vi "wavefront correction DMD control.vi"() -> ()   [LabVIEW 2016]
uses:
  <vilib>/DAQmx/write.llb/DAQmx Write (Analog DBL 1Chan 1Samp).vi
  <vilib>/DAQmx/read.llb/DAQmx Read (Analog 1D DBL 1Chan NSamp).vi
  <vilib>/Analysis/baseanly.llb/Mean (DBL).vi
  <vilib>/DAQmx/miscellaneous.llb/DAQmx Fill In Error Info.vi
  <vilib>/Analysis/NI_AALBase.lvlib
panel:
  out "Array":dbl[](array[numeric])
  out "1":dbl
  out "2":dbl
  out "3":dbl
  out "diff sq 3":dbl
  out "sum sq 3":dbl
  out "diff sq 2":dbl
  out "sq sum 2":dbl
  out "sum sq 1":dbl
  out "diff sq 1":dbl
  in  "t":dbl format="%#_13g"
  in  "Ignore \nthis mode":bool
  in  "Image Processing Methods":u16(ring) items=["mean", "Max Value", "sum of square", "diff square unit", "diff square"]
  out "WC finished":bool
  out "Project twice":bool
  out "Raw Data":dbl[](graph)
  out "evaluation value":dbl[](array[numeric])
  out "max index":i32
  in  "Y-Z Plane":bool
  out "Zernike index":i32
  in  "Num of Zernike Modes":dbl=3.0
  out "Real time Centre A":dbl=1.0
  out "Real time search gap":dbl
  out "unsigned 8bit integer":u8[][](array[numeric])
  out "Total Pack":dbl=6.0
  out "Hill-climbing \n   finished":bool
  in  "Ending search gap":dbl=0.05
  out "Zernike Coefficient":dbl[](array[numeric])=[0.0, 0.0, 1.0, 0.0, 0.0, 0.0, 0.0, 0.0, 0.0, 0.0, 0.0]
  in  "Start Centre A":dbl
  in  "Start search gap":dbl=0.4
  out "mean 2":dbl format="%0.2f"
  out "After oversampling-average 2":dbl[](graph)
  out "min value 2":dbl
  out "max value 2":dbl
  out "mean 1":dbl=-0.00018088652505750976 format="%0.2f"
  out "After oversampling-average 1":dbl[](graph)=[-0.0001987272925039077, -0.00015036376606842504, -0.00015036376637934116, -0.00017454552963234145, -0.0002551514075879374, -0.0001302122972688334, -0.00021887876244739687, -0.00018260611717117636, -0.00024709081919180694, -7.781847603481e-05, -0.0001826061167439524, -0.00021081817373790434, -0.00013021229598707122, -0.00014633347159563422, -0.00017454552892679263, -0.00016648494136330033, -0.00021887876204420295, -0.0001302122969271596, -0.00018260611748689937, -0.0001664849421136326, -9.796994613718705e-05, -0.0002470908198677353, -0.00015842435409453145, -9.393965164216052e-05, -0.00017857582297060024, -0.00022290905548974952, -0.00013424258995260602, -0.00018663641039229478, -0.00021081817384015146, -0.00019872729225545605, -0.0001624546480710753, -0.00025112111349446094, -0.00010200024064859927, -0.00010603053385410598, -0.00018663641175439846, -0.00019066670548701511, -0.00010603053392713635, -0.0002309696438184535, -8.9909357601442e-05, -0.0001785758229006333, -0.00021081817380142232, -0.00026321199426764555, -0.00012215170847929257, -0.00023903023104912573, -0.00019872729242518435, -0.00012618200296277008, -0.00017454552973023523, -0.00021484846861402935, -0.00020275758701047728, -0.00024306052590350124, -0.00018260611762661882, -0.00013021229705651406, -0.00015036376600609176, -0.0002430605253256984, -0.00023903023118351978, -0.0002349999370652512, -0.0002269393493190637, -0.00013424259002825932, -0.00014230317787017, -0.00019872729245131002, -0.0001261820028735292, -0.00010200023977950455, -0.0002148484685278861, -0.00021887876255904118, -0.00013827288524260415, -0.00019872729313313533, -0.0002148484685221406, -0.00014633347228160064, -0.00020275758639110144, -7.781847576089259e-05, -0.00014633347159867738, -0.00021081817366223055, -0.00021081817370487745, -0.00021484846775309002, -0.00010200023948238176, -0.00021484846837523008, -0.00015036376649324066, -0.0001584243542906475, -0.0002470908197968495, -0.0001261820032894319, -0.00025112111346112573, -0.00022290905618751688, -0.00015439405976456073, -0.00017857582285490896, -0.00015439405937578635, -0.00014633347152034754, -0.00016648494098961056, -0.0001423031779507158, -0.0002551514067878376, -0.0001261820028331801, -0.00020678788061648433, -0.0002753028768174787, -0.00014633347250696127, -0.0002551514074207985, -0.00015842435440751546, -0.00010200023968765957, -0.0002753028763261789, -0.00023096964359226534, -7.378818193678442e-05, -0.00016648494111095338, -0.00021887876158896606, -0.00013827288384506056, -0.0001826061166982094, -0.00021887876200616616, -0.0001705152354771987, -0.0001382728845284592, -0.00017857582385108457, -0.0001140911216208241, -0.00022693935036281564, -0.0002511211135111866, -0.00017454552965679386, -0.00011409112109491684, -0.0001946969986753396, -0.00015036376591257933, -0.0001946969982611868, -0.00020275758595170488, -0.0001503637655076617, -0.00014230317786099463, -0.00024306052517649937, -0.00010200023956235772, -0.0001503637662111079, -0.0001866364114763154, -0.00016648494235527059, -0.00019469699943921014, -0.0001584243542933623, -0.0001705152359230553, -0.00017454552938959368, -0.0002430605251173698, -0.00018663641049805447, -0.00022290905529435447, -0.00020678787978411914, -0.00021081817372709221, -9.796994534625098e-05, -0.00015036376607276814, -0.0002511211132029861, -0.00017051523611665082, -0.0001866364117673358, -0.00014633347284340956, -0.00017454552988072243, -0.00014633347230241984, -0.0001826061170662297, -0.00015842435359972182, -0.00018260611669343669, -0.0002551514064044735, -0.00021484846752859148, -0.00010200023891512827, -0.0002712725821161312, -0.00011812141476992442, -0.000122151709222508, -0.00016245464800623672, -0.00025515140743935576, -9.393965206130631e-05, -0.00016648494205608185, -0.00015842435428175614, -0.000158424354019495, -0.00019066670491674117, -0.00021081817402591077, -0.00010603053306169109, -0.0001463334716961554, -0.0001664849410222449, -0.00014633347173526376, -9.796994530323132e-05, -0.00021887876173339315, -0.0002994846397529397, -0.00020275758677174358, -0.00022693935021486926, -0.00023903023189267959, -0.00014633347248431497, -0.00024709081972418994, -0.00020275758672293496, -0.00016245464765312495, -0.00023903023114476115, -0.00020275758611747516, -0.0001866364105471905, -0.00019066670428520547, -0.0002511211126595155, -0.00021081817399597373, -0.00017051523534226194, -0.00022290905598825586, -0.00016245464789985017, -0.00020678788112111026, -0.00019469699917658138, -0.00017051523579818687, -0.00018260611736772357, -0.0002591817009361679, -0.00017454552936358266, -0.00017051523513136353, -0.00022290905536136475, -0.0001664849409539583, -0.00014633347152864118, -0.00013021229614974253, -0.00020678788014953778, -0.00011409112109187428, -0.00022290905621648625, -0.0001140911214072947, -7.378818290384523e-05, -0.00022290905660340472, -9.796994621100096e-05, -0.0001100608275008826, -0.00027127258258026184, -0.00020678788018434254, -0.00014230317786502345, -0.00013424258994523946, -0.00020678787979195971, -0.0002390302308507103, -0.0002470908188096414, -0.00031560581500641923, -0.00012215170885805348, -0.0002390302319484994, -0.00018260611748424968, -0.00017051523605180827, -0.00011409112149364246, -0.000206787880815561, -0.00011812141519833446, -0.00016648494149984909, -0.00011409112082213512, -0.0002067878800339049, -0.00015439405938788857, -0.00017857582274354006, -0.00012618200231082077, -0.00021081817402552892, -0.00023499993751946354, -0.00018663641111449909, -0.00017051523572419355, -0.00022693935041834674, -0.00020678788087198242, -0.00017857582364544665, -0.00021081817466581918, -0.00013827288456410468, -0.00013827288441875448, -0.0002309696432772496, -0.0002833634637586967, -0.00014633347163257721, -0.0002632119942615906, -0.0002632119943834941, -0.00023903023135536205, -0.00014633347203453652, -0.00021081817449440638, -0.00019469699931418246, -0.00014633347281451303, -0.00018663641146988893, -0.00021081817477948953, -0.00014230317877186632, -0.00023096964372758432, -0.00014633347201224554, -0.00017857582278618818, -0.00017857582265913937, -0.00018260611650596515, -0.00018663641039752316, -0.00018260611668388568, -0.0001302122963928654, -0.0002833634640793454, -0.00011006082762211242, -0.00022290905637235535, -0.00014633347261193422, -0.00023096964408310253, -0.00019469699912882273, -9.796994588552772e-05, -0.00017454552933081647, -0.00016245464744167696, -0.00015439405944757018, -0.00013424258994958362, -0.00022693934918768208, -0.0001423031778184172, -0.00017051523527400524, -0.00015842435371805848, -0.00021484846828916394, -0.00011409112157992023, -0.0003035149339342776, -0.00011812141551051005, -0.0001020002400533678, -0.00019469699918808032, -0.00013424259061247827, -6.572759429881741e-05, -0.00027933317003641576, -0.00021887876159123738, -0.00019872729205576374, -0.000174545528860661, -0.00022693934938217288, -0.0001463334719595995, -0.0001866364110829129, -0.00022693935006911405, -0.0002027575868808357, -0.0001624546480759602, -0.00022693935045359028, -0.00010603053366572733, -0.0002067878806376854, -0.00017857582330890143, -0.0001906667048355267, -0.00016648494132890412, -0.0001705152349730054, -0.0002390302308811581, -0.00016245464714889868, -0.0002753028759646651, -0.00012618200252910496, -0.00015439405975119133, -0.0001745455293896167, -0.00023096964417695983, -0.00010603053402439048, -0.0002672422893162719]
  out "min value 1":dbl=-0.00031560581500641923
  out "max value 1":dbl=-6.572759429881741e-05
  out "mean 3":dbl format="%0.2f"
  out "Frame 3":T1(plugin-control)
  out "Frame 1":T1(plugin-control)
  in  "A":dbl
  in  "ZerN":dbl
  in  "ZerM":dbl
  in  "Wavefront Correction":bool
  in  "Stop Imaging":bool
  in  "Ttrigger channels":tag="/Dev2/PFI0"
  in  "Counter":tag="Dev2/ctr0"
  in  "gain channels 2":tag="Dev2/ao0"
  out "actual triggere rate":dbl=20000.0
  out "SampClk.Rate 2":dbl=2000000.0
  in  "trigger rate 2":dbl=20000.0 format="%0.2p"
  in  "sampling rate 2":dbl=2000000.0
  in  "sample channels 2":tag="Dev2/ai0"
  out "Pixel number":dbl=10000.0
  out "Z number":dbl=1.0
  out "Y number":dbl=100.0
  out "X number":dbl=100.0
  in  "Num of per pack":i32=200
  in  "RangeZ":dbl=1.0
  in  "RangeY":dbl=30.0
  in  "RangeX":dbl=30.0
  in  "StepZ":dbl=1.0
  in  "StepY":dbl=0.3
  in  "StepX":dbl=0.3
  in  "CentreZ":dbl
  in  "CentreY":dbl
  in  "CentreX":dbl=38.0
  out "Error Out":errorcluster caption="error out"
  in  "Gain_Ch0":dbl(slide) scale=0.0..100.0
  out "After oversampling-average 3":dbl[](graph)
  in  "Start":i32=20
  in  "Auto Swing":bool=TRUE
  out "Frame 2":T1(plugin-control)
  in  "Swing 1":dbl(slide)=2.931034482758621 scale=0.0..5.0
  in  "Basis 1":dbl(slide)=0.46551724137931033 scale=-1.5..2.0
  out "max value 3":dbl
  out "min value 3":dbl
  in  "Delay time":u32=10 min=10 max=200
  out "# elements in queue":i32
  out "samples num 1":i32=30000
  out "Imaging":bool
  in  "image":bool
  out "Projecting":bool
  out "MATLAB script error":errorcluster
  out "DevAlloc":i32
  out "SerialNumber":i32=13271
  out "DeviceID":u32=173
  out "DMD Type":string="XGA"
  in  "Stop":bool
  out "ProjStartCont":i32
  in  "PictureTime/us":i32=48 min=0 max=256 step=1
  in  "Free pics":bool
  in  "Project":bool
  out "Idle":bool
  out "SeqAlloc":i32
  out "SequID":u32=4
  out "ErrorSeqPut":i32
  out "Progress":u8(slide)=33 scale=0.0..100.0
  out "Loading":bool
  in  "Load":bool
  out "No pics":bool=TRUE
  in  "Quit":bool
  out "PicNum":i32=10000
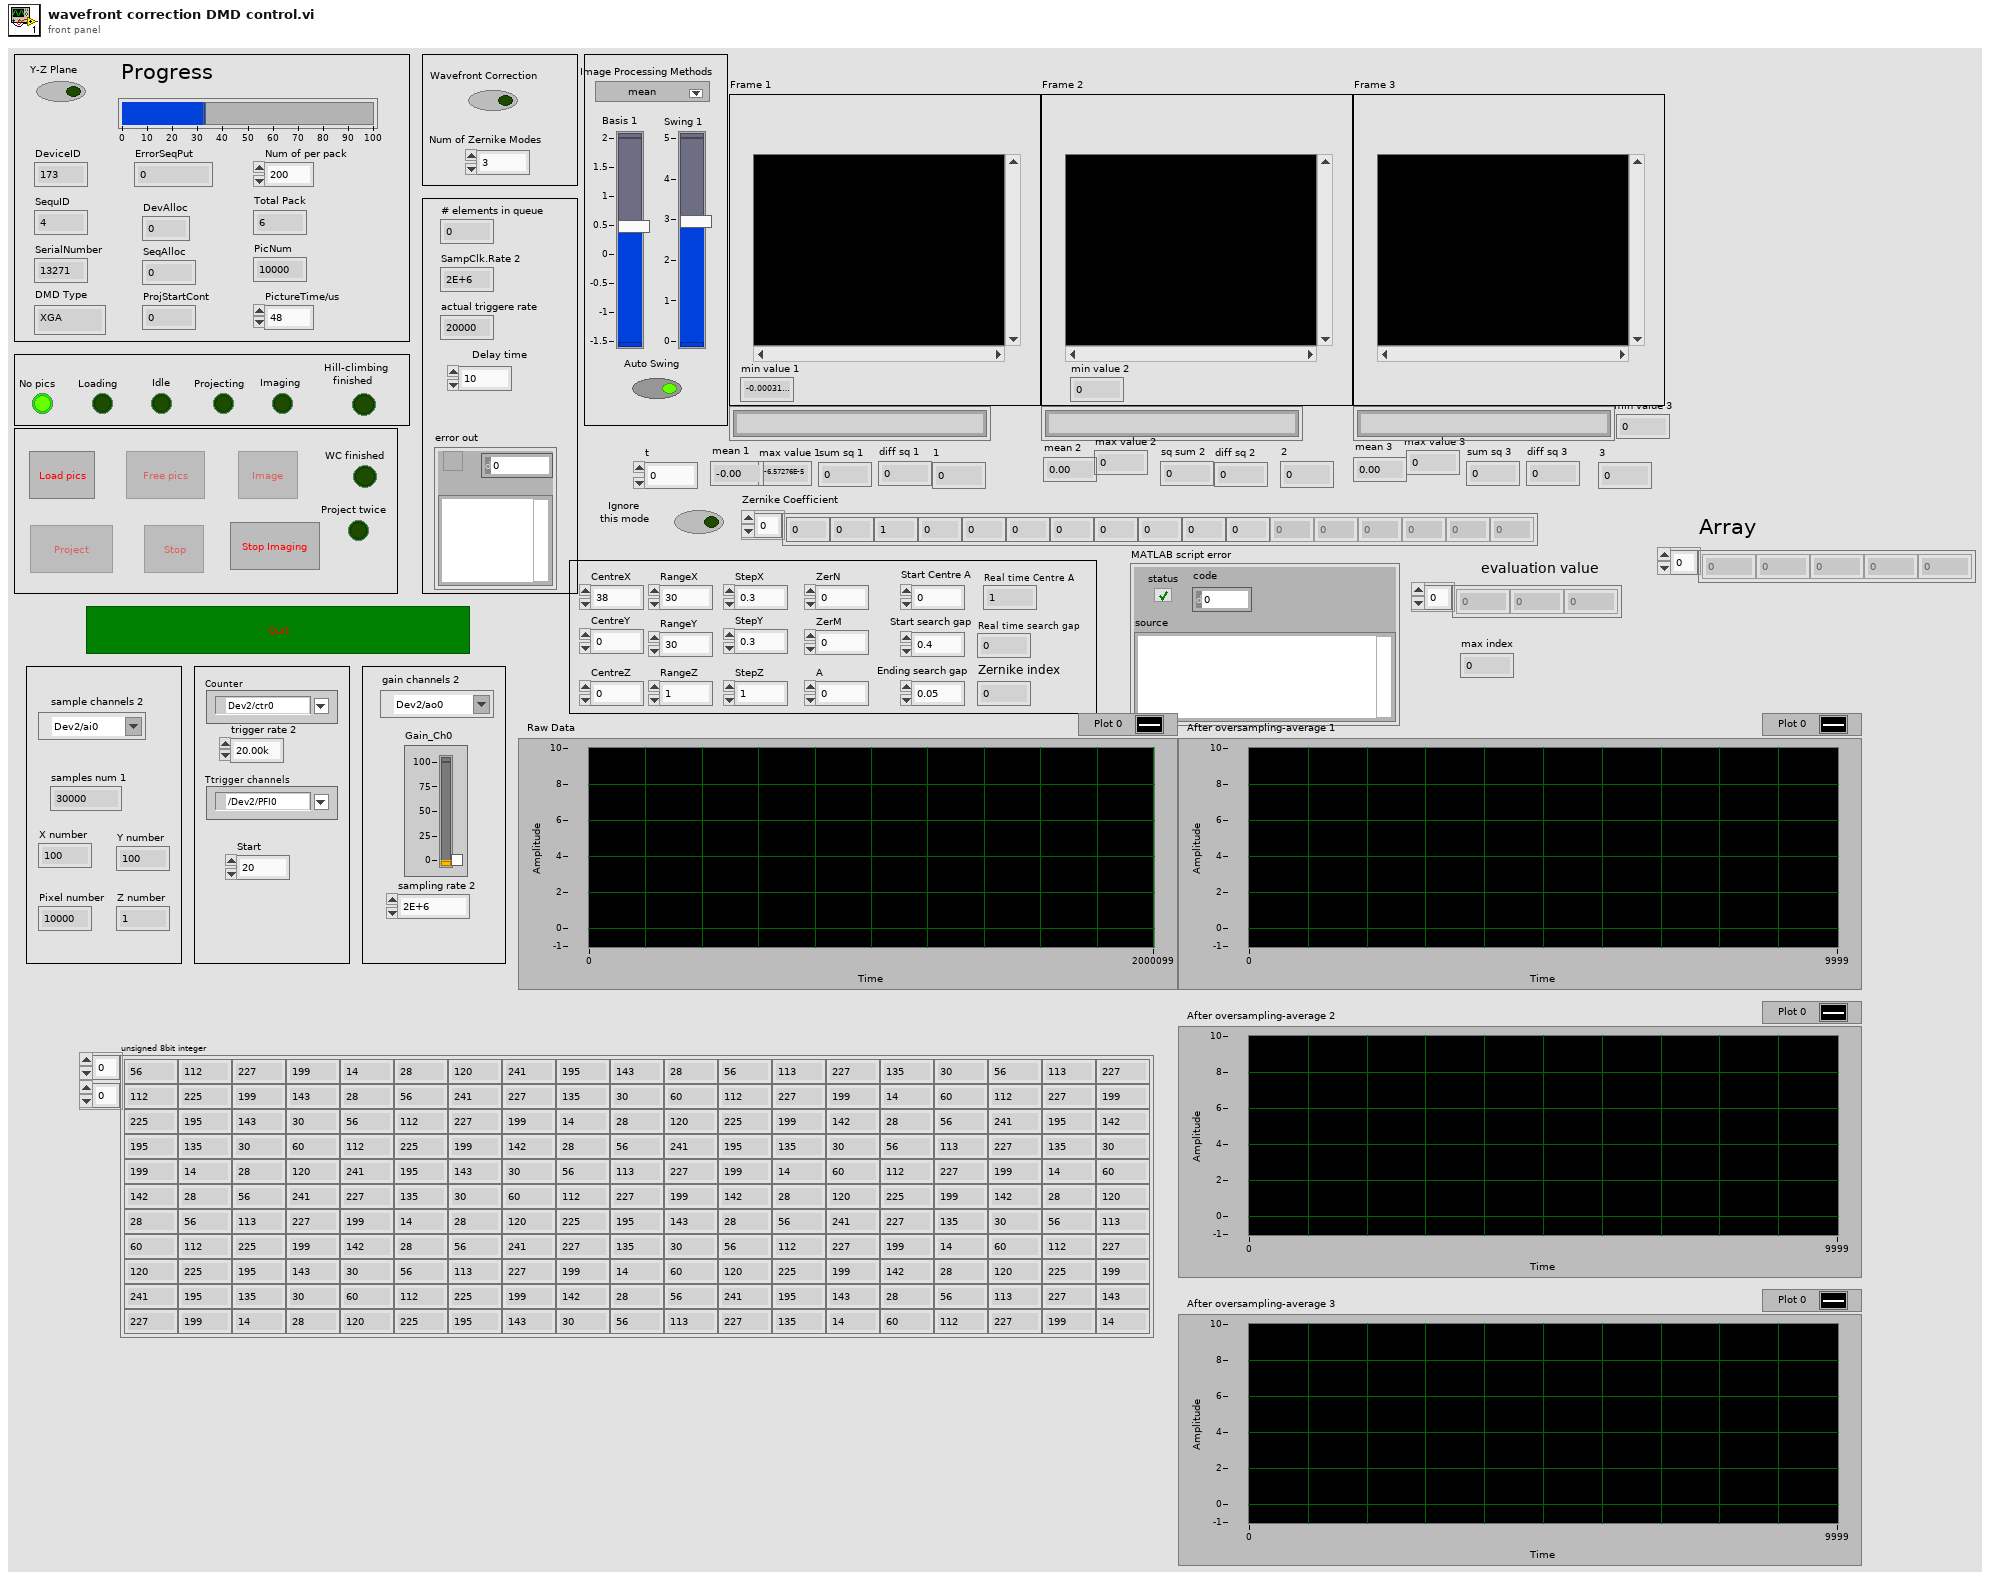
[diagram p1: front panel]
types:
  T1 = typedef "IMAQ Image.ctl" = refnum<image>
  T2 = enum16{"No sequence", "Load pics", "Idle", "Project", "Imaging", "Free pics"}
  T3 = enum8{"Enabled", "Disabled", "Disabled and Grayed Out"}
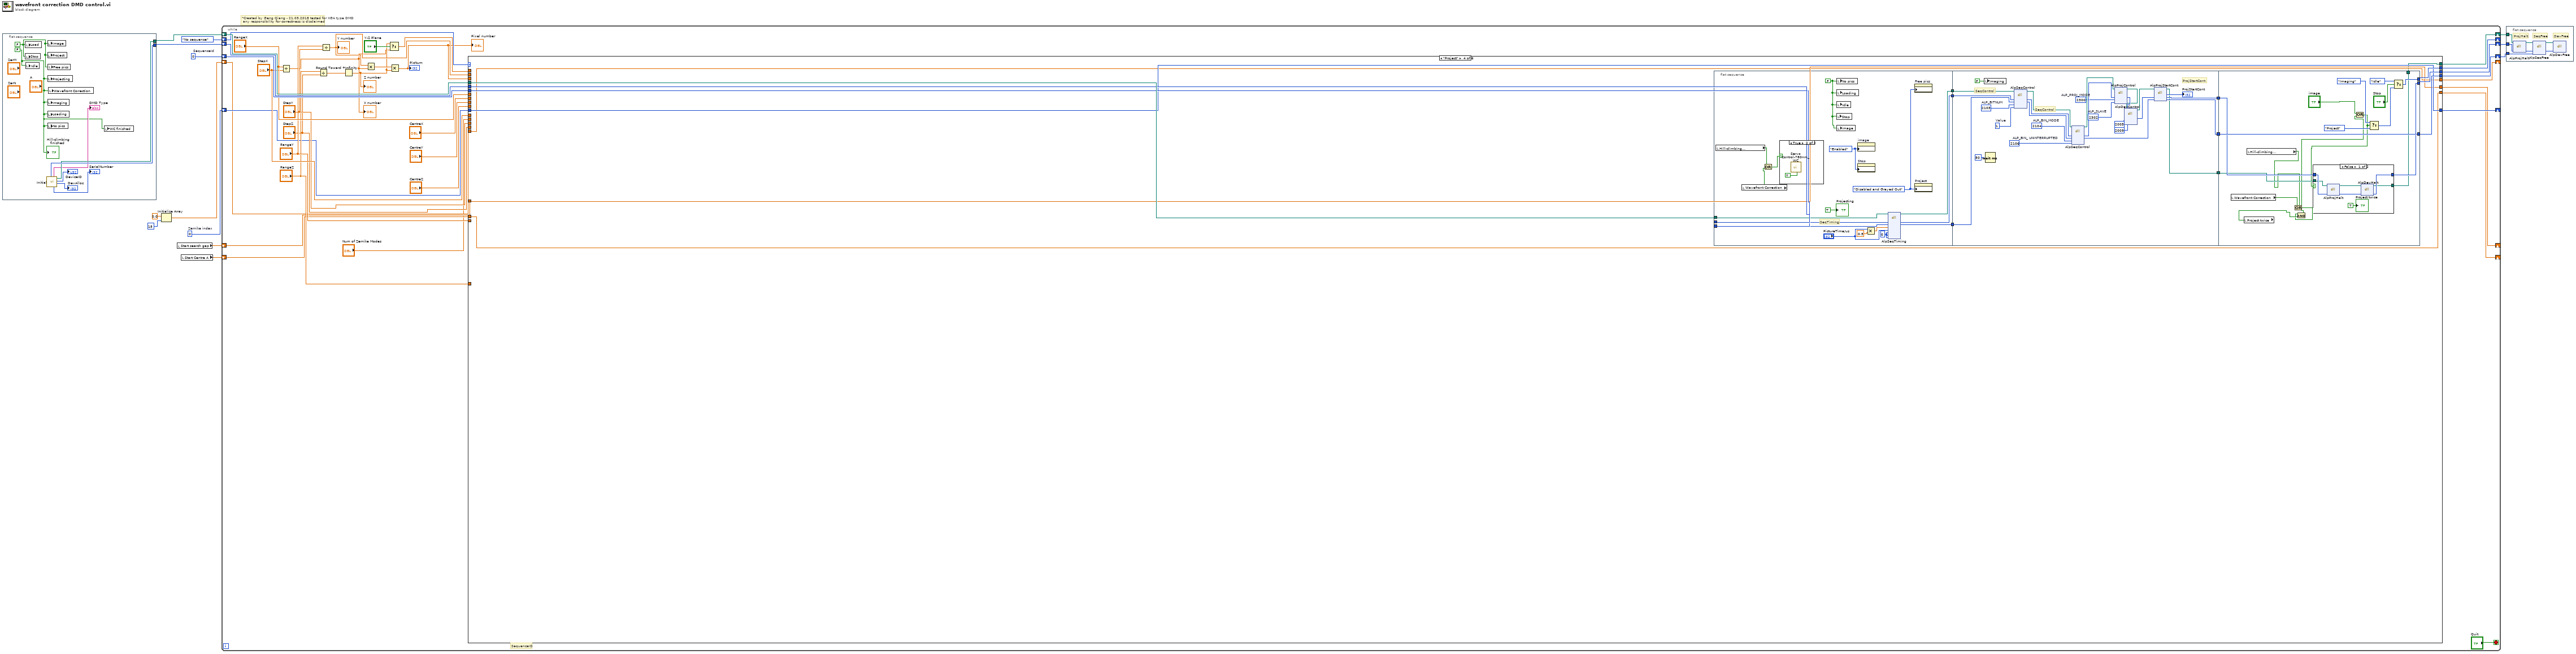
[diagram p0: block diagram]
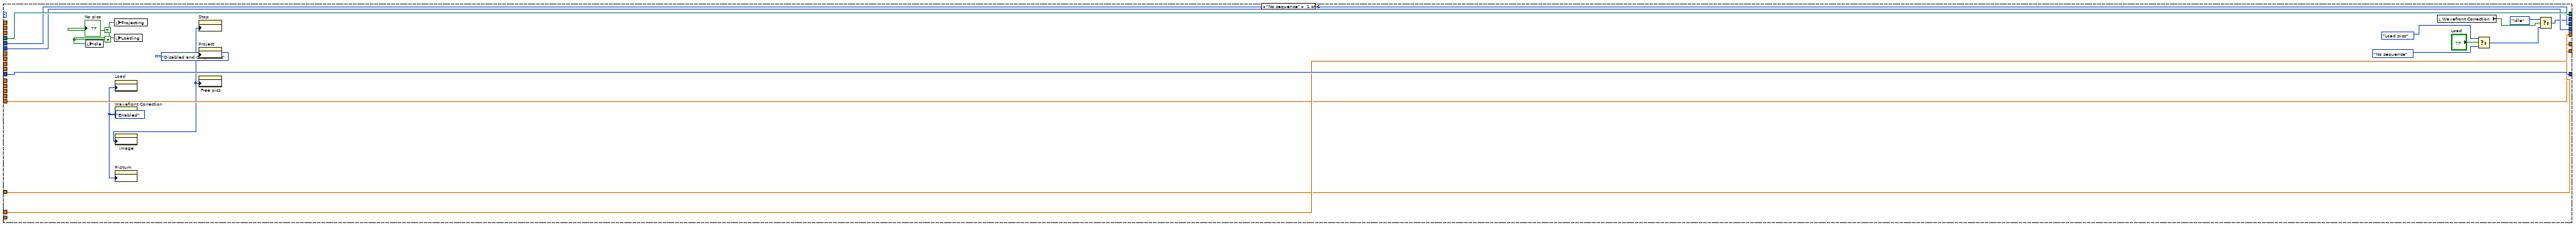
[diagram p2: hidden frame]
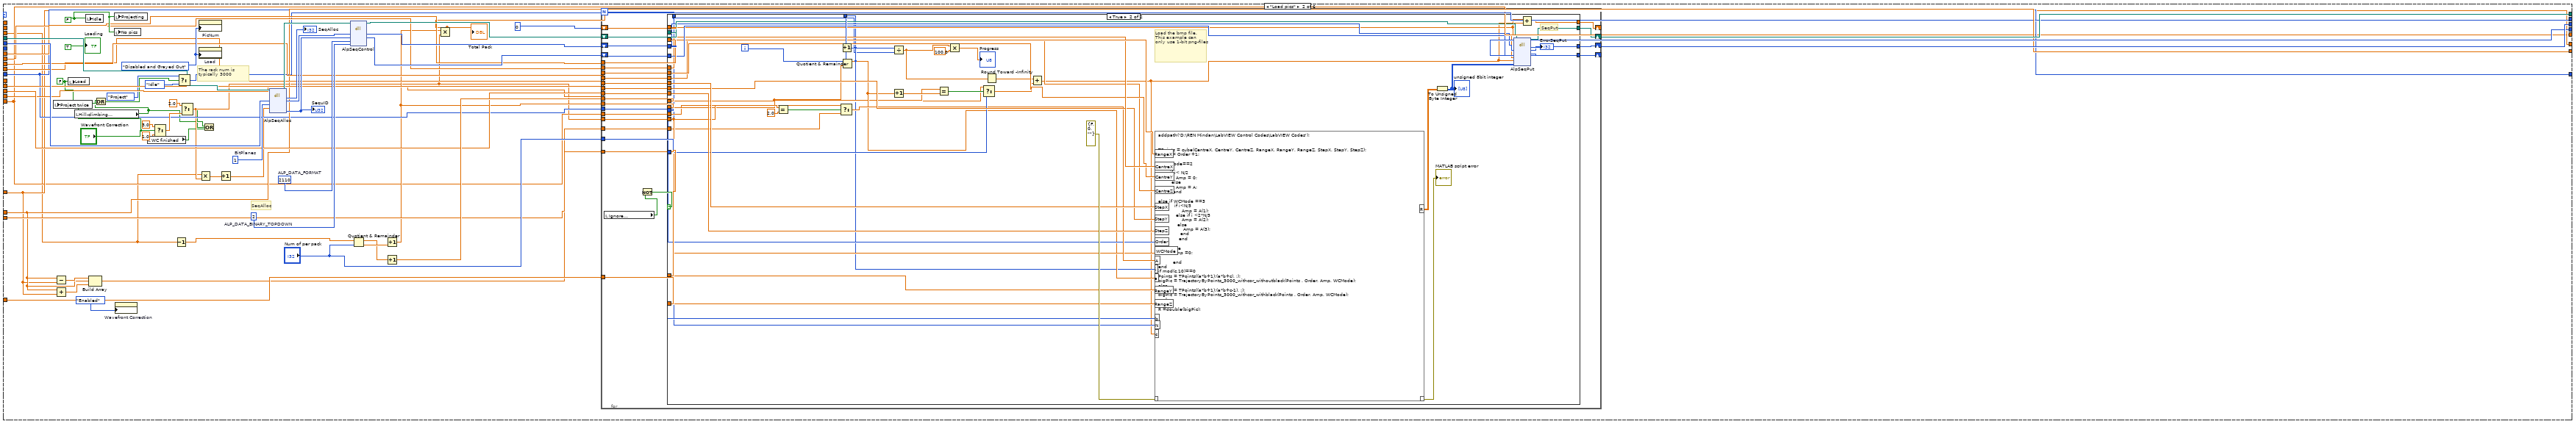
[diagram p3: hidden frame]
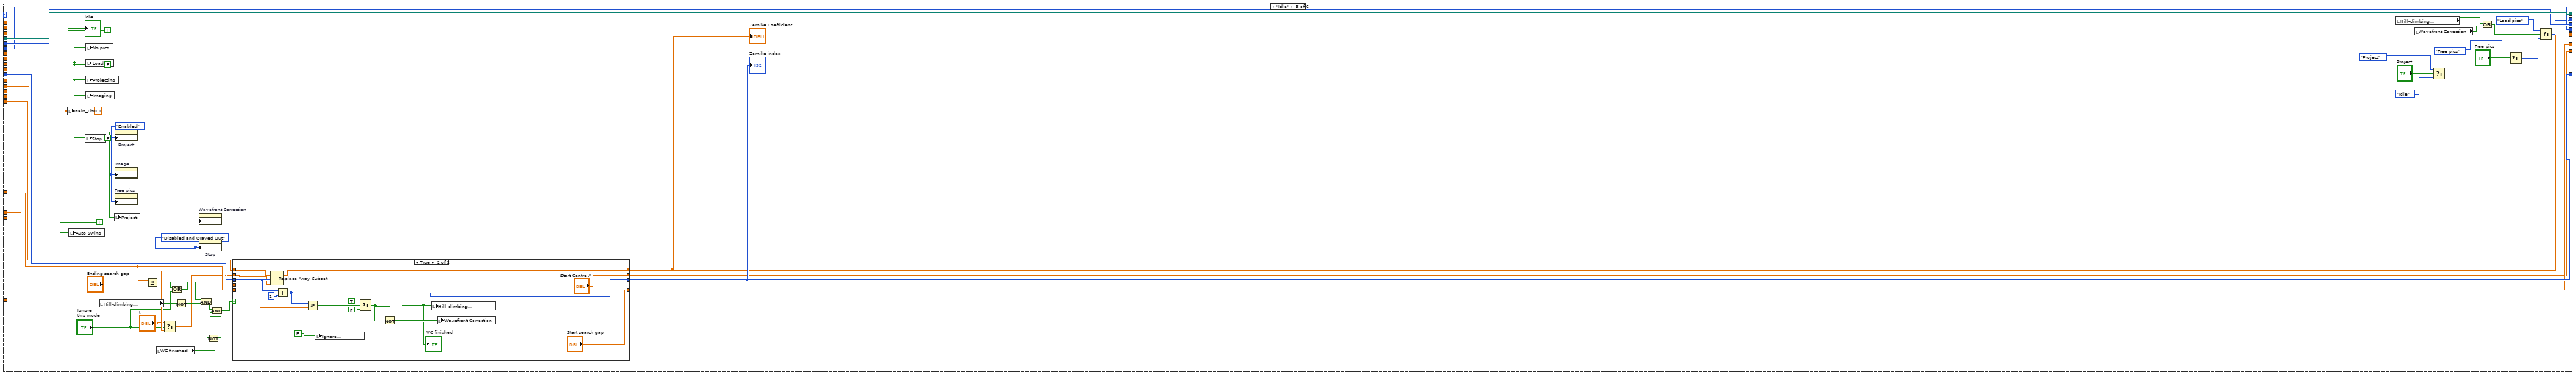
[diagram p5: hidden frame]
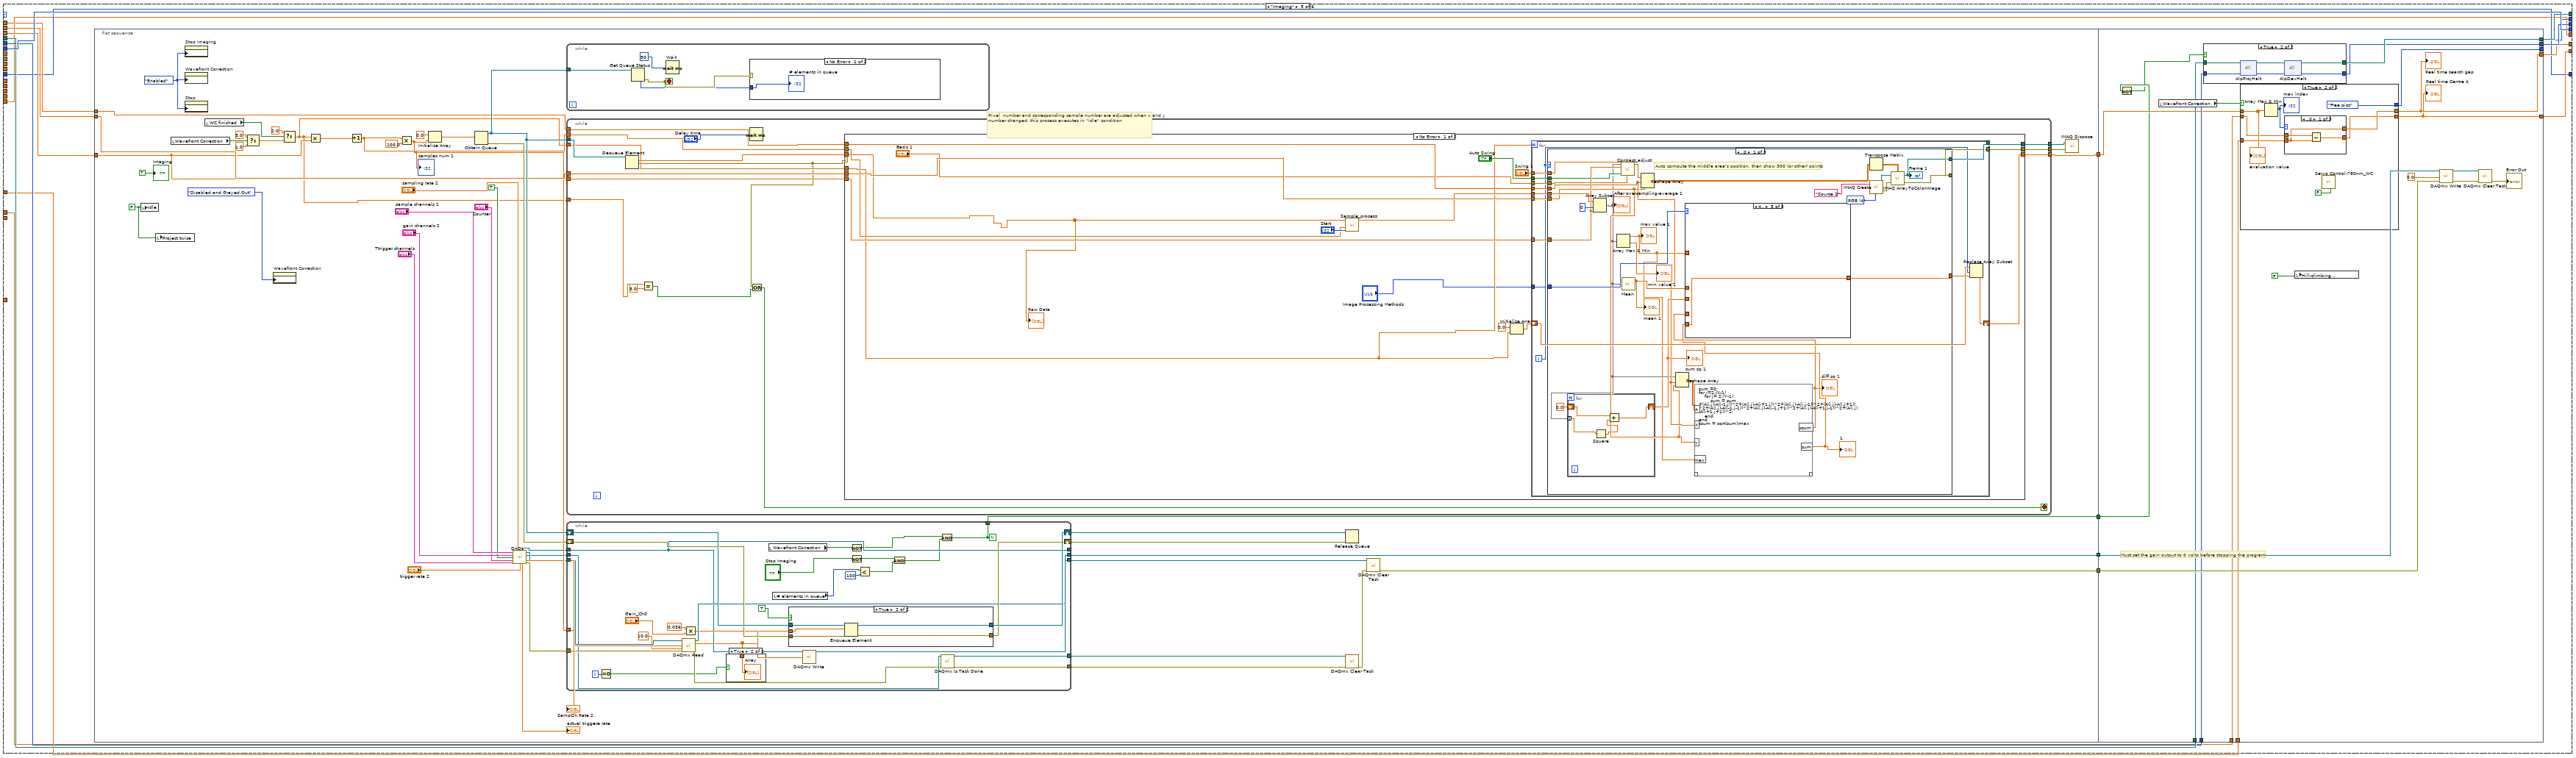
[diagram p9: hidden frame]
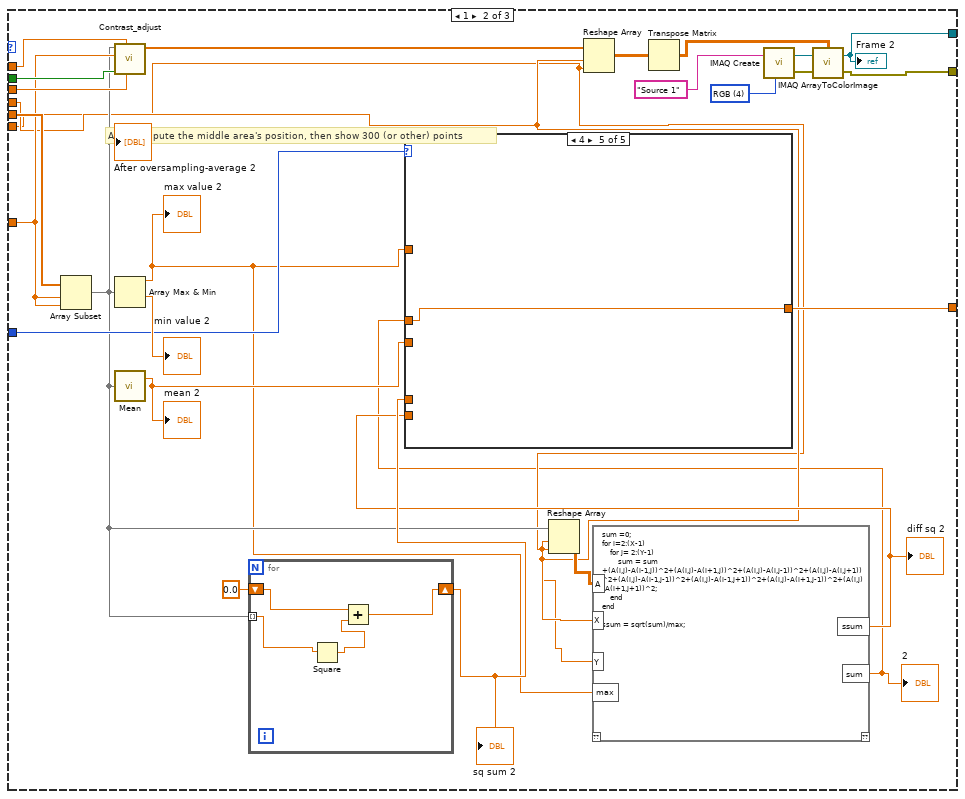
[diagram p14: hidden frame]
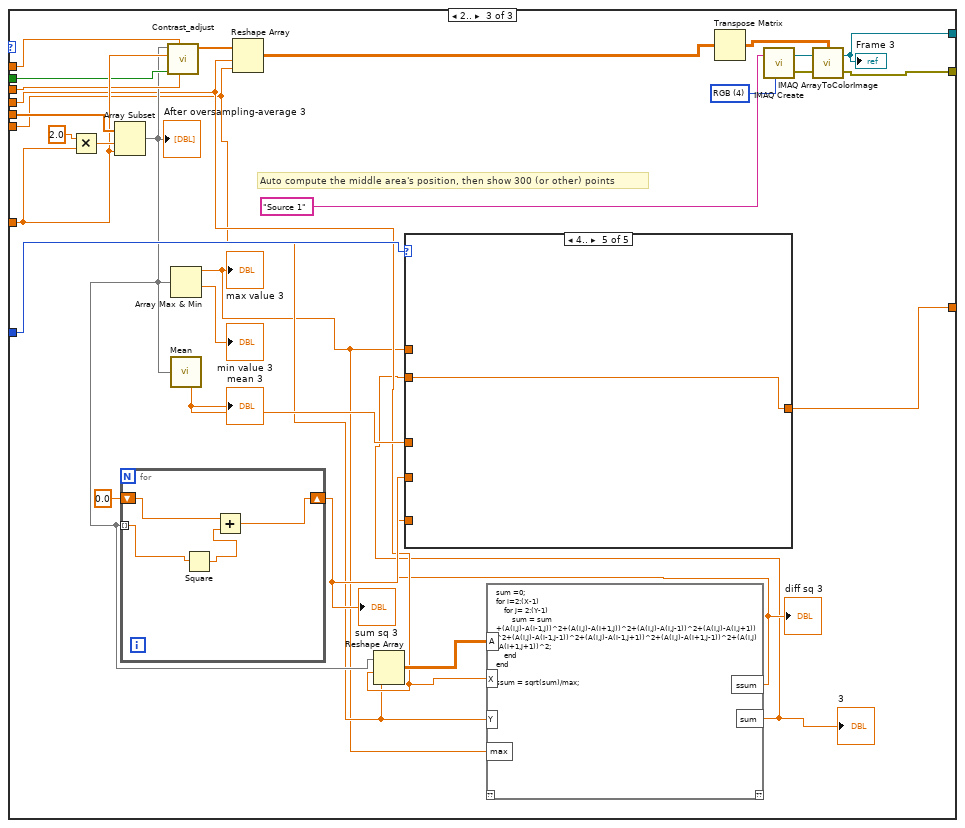
[diagram p19: hidden frame]
diagram:
  w6 = 0  # Zernike index
  w13 = u32 0  # SequenceId
  # "*Created by Geng Qiang - 21.03.2018 tested for XGA type DMD \n any responsibility for correctness is disclaimed"
  n1 = flat-sequence {
    tunnel: [w21] -> w12
    tunnel: [w20] -> w11
    frame #0 {
      w14 = FALSE ("load")
      w15 = FALSE ("load")
      n2 = local write "Load"(w15) -> ()
      n3 = local write "Stop"(w15) -> ()
      n4 = local write "Idle"(w14) -> ()
      n5 = call "Initial.vi"() -> ("DevAlloc"=→"DevAlloc":i32, "DeviceID"=→"DeviceID":u32, "path out"=w20:path, "SerialNumber"=→"SerialNumber":i32, "DMD Type"=→"DMD Type":string, "DeviceIdPtr"=w21:u32)  [unwired: 5 in, 1 out]
      n6 = local write "image"(w15) -> ()
      n7 = local write "Project"(w15) -> ()
      n8 = local write "Projecting"(w14) -> ()
      n9 = local write "Imaging"(w14) -> ()
      n10 = local write "Loading"(w14) -> ()
      n11 = local write "No pics"(w14) -> ()
      n12 = local write "Free pics"(w15) -> ()
      n13 = local write "Wavefront Correction"(w14) -> ()
      n14 = local write "WC finished"(w14) -> ()
      "Hill-climbing \n   finished" <- w14
    }
  }
  n15 = Initialize Array(0.0 ("element"), 15 ("dimension size")) -> (w2:dbl[])
  n16 = local read "Start search gap"() -> (w5:dbl)
  n17 = local read "Start Centre A"() -> (w4:dbl)
  n18 = while {
    shift-right: [w56] -> w10
    shift-left: w11 -> [w51]
    shift-right: [w55] -> w9
    shift-left: w12 -> [w52]
    shift-right: [w50] -> _
    shift-left: T2."No sequence" -> [w48]
    shift-right: [w53] -> w8
    shift-left: w13 -> [w54]
    shift-right: [w35] -> _
    shift-left: w6 -> [w36]
    shift-right: [w32] -> _
    shift-left: w5 -> [w34]
    shift-right: [w31] -> _
    shift-left: w4 -> [w33]
    shift-right: [w27] -> _
    shift-left: w2 -> [w28]
    stop <- "Quit" stop-if-true
    # "SequenceID"
    n19 = Divide(x="RangeX", y="StepX") -> (x/y=w24:dbl)
    "X number" <- w24
    n20 = Divide(x="RangeZ", y="StepZ") -> (x/y=w38:dbl)
    n21 = Divide(x="RangeY", y="StepY") -> (x/y=w37:dbl)
    "Y number" <- w37
    n22 = Round Toward +Infinity(x=w38) -> (ceil(x): smallest int >= x=w25:dbl)
    "Z number" <- w25
    n23 = Multiply(x=w37, y=w24) -> (x*y=w30:dbl)
    n24 = Select(t=w25, s="Y-Z Plane", f=w24) -> (s? t:f=w23:dbl)
    n25 = Multiply(x=w30, y=w25) -> (x*y=w29:dbl)
    "PicNum" <- w29
    "Pixel number" <- w29
    n26 = case shown="\"Project\"" w48 {
      tunnel: w51 -> [w74 w134 w253 w289 w374 w696]
      tunnel: w52 -> [w71 w133 w252 w287 w373 w695]
      tunnel: [w74 w119 w253 w273 w372 w693] -> w56
      tunnel: [w71 w121 w252 w283 w371 w691] -> w55
      tunnel: [w72 w120 w251 w282 w380 w692] -> w53
      tunnel: w54 -> [w72 _ w251 w286 w380 w694]
      tunnel: [w66 w95 w237 w281 w364 w686] -> w50
      tunnel: "RangeX" -> [_ w110 _ _ _ _]
      tunnel: "CentreY" -> [_ w108 _ _ _ _]
      tunnel: "CentreX" -> [_ w109 _ _ _ _]
      tunnel: "StepY" -> [_ w106 _ _ _ _]
      tunnel: "CentreZ" -> [_ w107 _ _ _ _]
      tunnel: "StepX" -> [_ w111 _ _ _ _]
      tunnel: "StepZ" -> [_ w105 _ _ _ _]
      tunnel: "RangeY" -> [_ w104 _ _ _ _]
      tunnel: "RangeZ" -> [_ w103 _ _ _ _]
      tunnel: w23 -> [_ _ _ _ w377 _]
      tunnel: w29 -> [_ w83 _ _ w376 _]
      tunnel: w37 -> [_ _ _ _ w375 _]
      tunnel: w36 -> [w62 w92 w236 w278 w365 w685]
      tunnel: [w62 w92 w235 w278 w365 w685] -> w35
      tunnel: w34 -> [w60 w89 w231 w277 w369 w684]
      tunnel: w33 -> [w61 w100 w220 w276 w366 w683]
      tunnel: [w60 w89 w233 w277 w368 w684] -> w32
      tunnel: [w61 w100 w232 w276 w367 w683] -> w31
      tunnel: w28 -> [w59 w88 w229 w275 w363 w682]
      tunnel: "Num of Zernike Modes" -> [_ _ w228 _ _ _]
      tunnel: [w59 w88 w227 w275 w363 w682] -> w27
      frame "No sequence" {
        w67 = FALSE ("No pics")
        w57 = T3."Disabled and Grayed Out" ("Disabled")
        w58 = T3."Enabled" ("Disabled")
        n27 = local write "Idle"(w67) -> ()
        n28 = local write "Projecting"(w67) -> ()
        n29 = local write "Loading"(w67) -> ()
        n30 = property on="Load" class="Bool (strict)"("DisabledEnum"=w58) -> ()  [unwired: 2 in, 2 out]
        n31 = property on="Wavefront Correction" class="Bool (strict)"("DisabledEnum"=w58) -> ()  [unwired: 2 in, 2 out]
        n32 = property on="image" class="Bool (strict)"("DisabledEnum"=w57) -> ()  [unwired: 2 in, 2 out]
        n33 = property on="PicNum" class="DigNum (strict)"("DisabledEnum"=w58) -> ()  [unwired: 2 in, 2 out]
        n34 = property on="Stop" class="Bool (strict)"("DisabledEnum"=w57) -> ()  [unwired: 2 in, 2 out]
        n35 = property on="Project" class="Bool (strict)"("DisabledEnum"=w57) -> ()  [unwired: 2 in, 2 out]
        n36 = property on="Free pics" class="Bool (strict)"("DisabledEnum"=w57) -> ()  [unwired: 2 in, 2 out]
        n37 = local read "Wavefront Correction"() -> (w63:bool)
        n38 = Select(t=T2."Load pics", s="Load", f=T2."No sequence") -> (s? t:f=w65:T2)
        n39 = Select(t=T2."Idle", s=w63, f=w65) -> (s? t:f=w66:T2)
        "No pics" <- TRUE ("No pics")
      }
      frame "Load pics" {
        w117 = FALSE ("Loading")
        w116 = T3."Disabled and Grayed Out" ("Disabled")
        w78 = FALSE ("load")
        w130 = 2  # ALP_DATA_BINARY_TOPDOWN
        w129 = 2110  # ALP_DATA_FORMAT
        w132 = 1  # BitPlanes
        # "The rack num is typically 3000"
        # "SeqAlloc"
        n40 = local write "Project twice"(w78) -> ()
        n41 = Subtract(x=w100, y=w89) -> (x-y=w101:dbl)
        n42 = Add(x=w100, y=w89) -> (x+y=w102:dbl)
        n43 = local write "Load"(w78) -> ()
        n44 = local read "Hill-climbing \n   finished"() -> (w76:bool)
        n45 = local write "Idle"(w117) -> ()
        n46 = Build Array(w101, w100, w102) -> (w81:dbl[])
        n47 = Or(x=w76, y="Wavefront Correction") -> (x .or. y?=w79:bool)
        n48 = local write "Projecting"(w117) -> ()
        n49 = local write "No pics"(w117) -> ()
        n50 = property on="Wavefront Correction" class="Bool (strict)"("DisabledEnum"=T3."Enabled" ("Disabled")) -> ()  [unwired: 2 in, 2 out]
        n51 = local read "WC finished"() -> (w77:bool)
        n52 = Select(t=3.0, s="Wavefront Correction", f=1.0) -> (s? t:f=w93:dbl)
        n53 = Decrement(x=w83) -> (x-1=w115:dbl)
        n54 = Select(t=T2."Project", s=w79, f=T2."Idle") -> (s? t:f=w95:T2)
        n55 = property on="PicNum" class="DigNum (strict)"("DisabledEnum"=w116) -> ()  [unwired: 2 in, 2 out]
        n56 = property on="Load" class="Bool (strict)"("DisabledEnum"=w116) -> ()  [unwired: 2 in, 2 out]
        n57 = Or(x=w76, y=w77) -> (x .or. y?=w75:bool)
        n58 = Select(t=2.0, s=w75, f=w93) -> (s? t:f=w84:dbl)
        n59 = Multiply(x=w83, y=w84) -> (x*y=w85:dbl)
        n60 = Increment(x=w85) -> (x+1=w82:dbl)
        n61 = dll-call lib="?" fn="AlpSeqAlloc"(path in=w134, "DeviceId"=w133, "BitPlanes"=w132, "PicNum"=w82) -> (path out=w127:path, "return type"=→"SeqAlloc":i32, "DeviceId"=w126:u32, "SequenceIdPtr"=w125:u32)  [unwired: 5 in, 1 out]
        "SequID" <- w125
        n62 = dll-call lib="?" fn="AlpSeqControl"(path in=w127, "DeviceId"=w126, "SequenceId"=w125, "ControlType"=w129, "ControlValue"=w130) -> (path out=w124:path, "DeviceId"=w123:u32, "SequenceId"=w122:u32)  [unwired: 5 in, 1 out]
        n63 = Quotient & Remainder(x=w115, y="Num of per pack") -> (x-y*floor(x/y)=w113:dbl, floor(x/y)=w128:dbl)
        n64 = Increment(x=w128) -> (x+1=w90:dbl)
        n65 = Increment(x=w113) -> (x+1=w112:dbl)
        n66 = Multiply(x=w90, y=w84) -> (x*y=w91:dbl)
        "Total Pack" <- w91
        n67 = for {
          N: w91 -> [w138]
          shift-right: [w161] -> w119
          shift-left: w124 -> [w162]
          shift-right: [w159] -> w121
          shift-left: w123 -> [w160]
          shift-right: [w157] -> w120
          shift-left: w122 -> [w158]
          tunnel: "Num of per pack" -> [w147]
          tunnel: w112 -> [w140]
          tunnel: w111 -> [w156]
          tunnel: w110 -> [w155]
          tunnel: w109 -> [w154]
          tunnel: w108 -> [w153]
          tunnel: w107 -> [w152]
          tunnel: w106 -> [w151]
          tunnel: w105 -> [w150]
          tunnel: w104 -> [w149]
          tunnel: w103 -> [w148]
          tunnel: w84 -> [w145]
          tunnel: w92 -> [w146]
          tunnel: w90 -> [w144]
          tunnel: w88 -> [w143]
          shift-right: [w141] -> _
          shift-left: 0 -> [w142]
          tunnel: w81 -> [w137]
          i -> [w139]
          n68 = local read "Ignore \nthis mode"() -> (w136:bool)
          n69 = Not(x=w136) -> (.not. x?=w135:bool)
          n70 = case shown="True" w135 {
            tunnel: w162 -> [w164 w209]
            tunnel: [w164 w208] -> w161
            tunnel: w160 -> [w166 w207]
            tunnel: [w166 w206] -> w159
            tunnel: w158 -> [w165 w205]
            tunnel: [w165 w204] -> w157
            tunnel: w156 -> [_ w197]
            tunnel: w155 -> [_ w196]
            tunnel: w154 -> [_ w195]
            tunnel: w153 -> [_ w194]
            tunnel: w152 -> [_ w193]
            tunnel: w151 -> [_ w192]
            tunnel: w150 -> [_ w191]
            tunnel: w149 -> [_ w190]
            tunnel: w148 -> [_ w189]
            tunnel: w147 -> [_ w187]
            tunnel: w146 -> [_ w183]
            tunnel: w145 -> [_ w182]
            tunnel: w144 -> [_ w180]
            tunnel: w143 -> [_ w179]
            tunnel: w142 -> [w163 w178]
            tunnel: [w163 w177] -> w141
            tunnel: w140 -> [_ w175]
            tunnel: w139 -> [_ w174]
            tunnel: w138 -> [_ w173]
            tunnel: w137 -> [_ w167]
            frame False {
            }
            frame True {
              # "Load the bmp file.\nThis example can \nonly use 1-bit png-files"
              # "SeqPut"
              n71 = Equal?(x=w182, y=2.0) -> (x = y?=w184:bool)
              n72 = Select(t=w179, s=w184, f=w167) -> (s? t:f=w186:dbl[])
              n73 = Increment(x=w174) -> (x+1=w172:i32)
              n74 = Quotient & Remainder(x=w174, y=w180) -> (x-y*floor(x/y)=w181:dbl)  [unwired: 1 out]
              n75 = Divide(x=w172, y=w173) -> (x/y=w171:dbl)
              n76 = Increment(x=w181) -> (x+1=w202:dbl)
              n77 = Equal?(x=w180, y=w202) -> (x = y?=w203:bool)
              n78 = Multiply(x=w171, y=100.0) -> (x*y=→"Progress":dbl)
              n79 = Select(t=w175, s=w203, f=w187) -> (s? t:f=w170:dbl)
              n80 = Round Toward -Infinity(1:w171) -> (0:w169:dbl)
              n81 = Add(x=w169, y=w170) -> (x+y=w168:dbl)
              n82 = script code="addpath('D:\\REN Mindan\\LabVIEW Control Codes\\LabVIEW Codes');\n\n\nTPoints = cube(CentreX, CentreY, CentreZ, RangeX, RangeY, RangeZ, StepX, StepY, StepZ);\nOrder = Order +1;\n\nif WCMode==2\n     \n        if i< N/2\n            Amp = 0;\n         else\n            Amp = A;\n          end\n       \nelse if WCMode ==3\n           if i<N/3\n                Amp = A(1);\n            else if i <2*N/3\n                Amp = A(2);\n             else\n                 Amp = A(3);\n               end\n              end\n        \n         else \n          Amp =0;\n          \n          end\nend\nif mod(c,10)==0\nPoints = TPoints((a*b+1):(a*b+c), :);\nbigPic = TrajectoryByPoints_3000_withcor_withoutblack(Points , Order, Amp, WCMode);\nelse \nPoints = TPoints((a*b+1):(a*b+c-1), :);\nbigPic = TrajectoryByPoints_3000_withcor_withblack(Points , Order, Amp, WCMode);\nend\n\nR =double(bigPic);"("??"=errorcluster {"status"=FALSE, "code"=0, "source"=""} ("error in"), "CentreX"=w195, "CentreY"=w194, "CentreZ"=w193, "StepX"=w197, "StepY"=w192, "StepZ"=w191, "Order"=w183, "RangeX"=w196, "RangeY"=w190, "RangeZ"=w189, "a"=w181, "b"=w187, "c"=w168, "A"=w186, "WCMode"=w182, "i"=w174, "N"=w173) -> ("??"=→"MATLAB script error":errorcluster, "R"=w188:dbl[][])
              n83 = To Unsigned Byte Integer(number=w188) -> (unsigned 8bit integer=w176:u8[][])
              "unsigned 8bit integer" <- w176
              n84 = dll-call lib="?" fn="AlpSeqPut"(path in=w209, "DeviceId"=w207, "SequenceId"=w205, "PicOffset"=w178, "PicLoad"=w168, "UserArrayPtr"=w176) -> (path out=w208:path, "return type"=→"ErrorSeqPut":i32, "DeviceId"=w206:u32, "SequenceId"=w204:u32)  [unwired: 5 in, 1 out]
              n85 = Add(x=w178, y=w168) -> (x+y=w177:dbl)
            }
          }
        }
        "Loading" <- TRUE ("Loading")
      }
      frame "Idle" {
        w226 = FALSE ("Loading")
        w230 = T3."Disabled and Grayed Out" ("Disabled")
        w240 = T3."Enabled" ("Disabled")
        w241 = FALSE ("stop")
        n86 = local write "Gain_Ch0"(0.0 ("Gain_Ch0")) -> ()
        n87 = local write "Auto Swing"(TRUE ("Scanning")) -> ()
        n88 = local write "Stop"(w241) -> ()
        n89 = local write "No pics"(w226) -> ()
        n90 = local write "Loading"(w226) -> ()
        n91 = local write "Projecting"(w226) -> ()
        n92 = local write "Imaging"(w226) -> ()
        n93 = local read "Hill-climbing \n   finished"() -> (w225:bool)
        n94 = local write "Project"(w241) -> ()
        n95 = property on="Project" class="Bool (strict)"("DisabledEnum"=w240) -> ()  [unwired: 2 in, 2 out]
        n96 = property on="image" class="Bool (strict)"("DisabledEnum"=w240) -> ()  [unwired: 2 in, 2 out]
        n97 = property on="Free pics" class="Bool (strict)"("DisabledEnum"=w240) -> ()  [unwired: 2 in, 2 out]
        n98 = Less Or Equal?(x=w231, y="Ending search gap") -> (x <= y?=w216:bool)
        n99 = local read "WC finished"() -> (w214:bool)
        n100 = Select(t="t", s="Ignore \nthis mode", f=w220) -> (s? t:f=w218:dbl)
        n101 = Or(x=w216, y="Ignore \nthis mode") -> (x .or. y?=w217:bool)
        n102 = Not(x=w225) -> (.not. x?=w224:bool)
        n103 = property on="Wavefront Correction" class="Bool (strict)"("DisabledEnum"=w230) -> ()  [unwired: 2 in, 2 out]
        n104 = property on="Stop" class="Bool (strict)"("DisabledEnum"=w230) -> ()  [unwired: 2 in, 2 out]
        n105 = And(x=w217, y=w224) -> (x .and. y?=w213:bool)
        n106 = Not(x=w214) -> (.not. x?=w212:bool)
        n107 = And(x=w213, y=w212) -> (x .and. y?=w211:bool)
        n108 = case shown="True" w211 {
          tunnel: w236 -> [w257 w270]
          tunnel: [w257 w271] -> w235
          tunnel: w218 -> [w255 w259]
          tunnel: [w256 "Start search gap"] -> w233
          tunnel: [w255 "Start Centre A"] -> w232
          tunnel: w231 -> [w256 _]
          tunnel: w229 -> [w254 w263]
          tunnel: w228 -> [_ w262]
          tunnel: [w254 w261] -> w227
          frame False {
          }
          frame True {
            n109 = Replace Array Subset(array=w263, new element=w259, index=w270) -> (w261:dbl[])
            n110 = Add(x=w270, y=1) -> (x+y=w271:i32)
            n111 = Greater Or Equal?(x=w271, y=w262) -> (x >= y?=w267:bool)
            n112 = local write "Ignore \nthis mode"(FALSE) -> ()
            n113 = Select(t=TRUE, s=w267, f=FALSE) -> (s? t:f=w260:bool)
            "WC finished" <- w260
            n114 = Not(x=w260) -> (.not. x?=w264:bool)
            n115 = local write "Hill-climbing \n   finished"(w260) -> ()
            n116 = local write "Wavefront Correction"(w264) -> ()
          }
        }
        "Zernike index" <- w235
        "Zernike Coefficient" <- w227
        n117 = local read "Hill-climbing \n   finished"() -> (w221:bool)
        n118 = local read "Wavefront Correction"() -> (w223:bool)
        n119 = Select(t=T2."Project", s="Project", f=T2."Idle") -> (s? t:f=w249:T2)
        n120 = Or(x=w221, y=w223) -> (x .or. y?=w222:bool)
        n121 = Select(t=T2."Free pics", s="Free pics", f=w249) -> (s? t:f=w239:T2)
        n122 = Select(t=T2."Load pics", s=w222, f=w239) -> (s? t:f=w237:T2)
        "Idle" <- TRUE ("Idle")
      }
      frame "Project" {
        n123 = flat-sequence {
          tunnel: w289 -> [w302]
          tunnel: [w301] -> w288
          tunnel: w287 -> [w300]
          tunnel: w286 -> [w299]
          tunnel: [w298] -> w285
          tunnel: [w297] -> w284
          tunnel: [w324] -> w280
          tunnel: w288 -> [w328]
          tunnel: w285 -> [w327]
          tunnel: w284 -> [w326]
          tunnel: [w325] -> w279
          tunnel: [w314] -> w274
          tunnel: w280 -> [w346]
          tunnel: [w345] -> w283
          tunnel: [w352] -> w282
          tunnel: w279 -> [w352]
          tunnel: [w348] -> w281
          tunnel: w274 -> [w344]
          tunnel: [w343] -> w273
          frame #0 {
            w293 = FALSE ("Projecting")
            w294 = T3."Enabled" ("Disabled")
            w296 = T3."Disabled and Grayed Out" ("Disabled")
            w305 = 0 ("element")
            # "SeqTiming"
            n124 = local read "Hill-climbing \n   finished"() -> (w292:bool)
            n125 = local read "Wavefront Correction"() -> (w291:bool)
            n126 = Or(x=w292, y=w291) -> (x .or. y?=w290:bool)
            n127 = case shown="True" w290 {
              frame False {
              }
              frame True {
                n128 = call "Servo Control-780nm_WC.vi"("DMD Shutter"=TRUE) -> ()  [unwired: 11 in]
              }
            }
            n129 = local write "Stop"(w293) -> ()
            n130 = local write "No pics"(w293) -> ()
            n131 = local write "Loading"(w293) -> ()
            n132 = local write "Idle"(w293) -> ()
            n133 = local write "image"(w293) -> ()
            n134 = property on="image" class="Bool (strict)"("DisabledEnum"=w294) -> ()  [unwired: 2 in, 2 out]
            n135 = property on="Stop" class="Bool (strict)"("DisabledEnum"=w294) -> ()  [unwired: 2 in, 2 out]
            n136 = Multiply(x="PictureTime/us", y=0.5) -> (x*y=w306:dbl)
            n137 = dll-call lib="C:/Users/CHEN Lab WorkStation/Desktop/LabVIEW Control Codes/alp4395.dll" fn="AlpSeqTiming"(path in=w302, "DeviceId"=w300, "SequenceId"=w299, "IlluminateTime"=w306, "PictureTime"="PictureTime/us", "TriggerDelay"=w305, "TriggerPulseWidth"=w305, "VdDelay"=w305) -> (path out=w301:path, "DeviceId"=w298:u32, "SequenceId"=w297:u32)  [unwired: 8 in, 1 out]
            n138 = property on="Free pics" class="Bool (strict)"("DisabledEnum"=w296) -> ()  [unwired: 2 in, 2 out]
            n139 = property on="Project" class="Bool (strict)"("DisabledEnum"=w296) -> ()  [unwired: 2 in, 2 out]
            "Projecting" <- TRUE ("Projecting")
          }
          frame #1 {
            w320 = u32 2302  # ALP_SLAVE
            w321 = 2300  # ALP_PROJ_MODE
            w333 = 2106  # ALP_BIN_ UNINTERRUPTED
            w332 = 2104  # ALP_BIN_MODE
            w331 = 1  # Value
            w330 = 2103  # ALP_BITNUM
            # "SeqControl"
            # "ProjStartCont"
            # "SeqControl"
            n140 = local write "Imaging"(FALSE ("Project")) -> ()
            n141 = Wait (ms)(milliseconds to wait=u32 50) -> ()  [unwired: 1 out]
            n142 = dll-call lib="C:/Users/CHEN Lab WorkStation/Desktop/LabVIEW Control Codes/alp4395.dll" fn="AlpSeqControl"(path in=w328, "DeviceId"=w327, "SequenceId"=w326, "ControlType"=w330, "ControlValue"=w331) -> (path out=w319:path, "DeviceId"=w318:u32, "SequenceId"=w317:u32)  [unwired: 5 in, 1 out]
            n143 = dll-call lib="C:/Users/CHEN Lab WorkStation/Desktop/LabVIEW Control Codes/alp4395.dll" fn="AlpSeqControl"(path in=w319, "DeviceId"=w318, "SequenceId"=w317, "ControlType"=w332, "ControlValue"=w333) -> (path out=w323:path, "DeviceId"=w322:u32, "SequenceId"=w316:u32)  [unwired: 5 in, 1 out]
            n144 = dll-call lib="C:/Users/CHEN Lab WorkStation/Desktop/LabVIEW Control Codes/alp4395.dll" fn="AlpProjControl"(path in=w323, "DeviceId"=w322, "ControlType"=w321, "ControlValue"=w320) -> (path out=w309:path, "DeviceId"=w313:u32)  [unwired: 5 in, 1 out]
            n145 = dll-call lib="C:/Users/CHEN Lab WorkStation/Desktop/LabVIEW Control Codes/alp4395.dll" fn="AlpDevControl"(path in=w309, "DeviceId"=w313, "ControlType"=2005, "ControlValue"=u32 2009) -> (path out=w308:path, "DeviceId"=w312:u32)  [unwired: 5 in, 1 out]
            n146 = dll-call lib="C:/Users/CHEN Lab WorkStation/Desktop/LabVIEW Control Codes/alp4395.dll" fn="AlpProjStartCont" ("alpD40.dll:AlpProjStart")(path in=w308, "DeviceId"=w312, "SequenceId"=w316) -> (path out=w314:path, "return type"=→"ProjStartCont":i32, "DeviceId"=w324:u32, "SequenceId"=w325:u32)  [unwired: 2 in, 1 out]
          }
          frame #2 {
            n147 = local read "Wavefront Correction"() -> (w338:bool)
            n148 = local read "Project twice"() -> (w341:bool)
            n149 = local read "Hill-climbing \n   finished"() -> (w339:bool)
            n150 = Or(x=w339, y=w338) -> (x .or. y?=w337:bool)
            n151 = And(x=w337, y=w341) -> (x .and. y?=w336:bool)
            n152 = Or(x="image", y=w336) -> (x .or. y?=w335:bool)
            n153 = case shown="False" w335 {
              tunnel: w346 -> [w357 w361]
              tunnel: [w356 w361] -> w345
              tunnel: w344 -> [w355 w360]
              tunnel: [w354 w360] -> w343
              frame False {
                n154 = dll-call lib="D:/documents/Dropbox/Only me/wavefront_correction/LabVIEW Control Codes/LabVIEW Codes/alp4395.dll" fn="AlpProjHalt"(path in=w355, "DeviceId"=w357) -> (path out=w359:path, "DeviceId"=w358:u32)  [unwired: 3 in, 1 out]
                n155 = dll-call lib="D:/documents/Dropbox/Only me/wavefront_correction/LabVIEW Control Codes/LabVIEW Codes/alp4395.dll" fn="AlpDevHalt"(path in=w359, "DeviceId"=w358) -> (path out=w354:path, "DeviceId"=w356:u32)  [unwired: 3 in, 1 out]
                "Project twice" <- TRUE ("Project twice")
              }
              frame True {
              }
            }
            n156 = Select(t=T2."Imaging", s=w335, f=T2."Project") -> (s? t:f=w347:T2)
            n157 = Select(t=T2."Idle", s="Stop", f=w347) -> (s? t:f=w348:T2)
          }
        }
      }
      frame "Imaging" {
        n158 = flat-sequence {
          tunnel: [w415] -> w379
          tunnel: [w414] -> w378
          tunnel: w377 -> [w413]
          tunnel: w376 -> [w385]
          tunnel: w375 -> [w412]
          tunnel: [w396] -> w370
          tunnel: [w384] -> w362
          tunnel: w379 -> [w647]
          tunnel: w378 -> [w648]
          tunnel: w374 -> [w646]
          tunnel: w373 -> [w645]
          tunnel: [w644] -> w372
          tunnel: [w643] -> w371
          tunnel: w370 -> [w642]
          tunnel: w369 -> [w638]
          tunnel: [w641] -> w368
          tunnel: [w640] -> w367
          tunnel: w366 -> [w639]
          tunnel: [w636] -> w364
          tunnel: w362 -> [w635]
          frame #0 {
            w383 = FALSE
            w395 = T3."Enabled" ("Disabled")
            # "Pixel  number and corresponding sample number are adjusted when x and y number changed, this process executes in \"idle\" condition"
            n159 = local write "Idle"(w383) -> ()
            n160 = local write "Project twice"(w383) -> ()
            n161 = local read "Wavefront Correction"() -> (w391:bool)
            n162 = property on="Stop Imaging" class="Bool (strict)"("DisabledEnum"=w395) -> ()  [unwired: 2 in, 2 out]
            n163 = property on="Wavefront Correction" class="Bool (strict)"("DisabledEnum"=w395) -> ()  [unwired: 2 in, 2 out]
            n164 = property on="Stop" class="Bool (strict)"("DisabledEnum"=w395) -> ()  [unwired: 2 in, 2 out]
            n165 = local read "WC finished"() -> (w388:bool)
            n166 = Select(t=3.0, s=w391, f=1.0) -> (s? t:f=w392:dbl)
            n167 = property on="Wavefront Correction" class="Bool (strict)"("DisabledEnum"=T3."Disabled and Grayed Out" ("Disabled")) -> ()  [unwired: 2 in, 2 out]
            n168 = Select(t=2.0, s=w388, f=w392) -> (s? t:f=w382:dbl)
            n169 = Multiply(x=w382, y=w385) -> (x*y=w386:dbl)
            n170 = Increment(x=w386) -> (x+1=w394:dbl)
            n171 = Multiply(x=w394, y=100.0) -> (x*y=w410:dbl)
            "samples num 1" <- w410
            n172 = Initialize Array(0.0 ("element"), w410) -> (w421:dbl[])
            n173 = Obtain Queue(element data type=w421) -> (queue out=w423:refnum<queue>, error out=w427:errorcluster)  [unwired: 4 in, 1 out]
            n174 = call "DAQs.vi"("sample channels"="sample channels 2", "rate"="sampling rate 2", "gain channels"="gain channels 2", "Sync or not"=TRUE, "Counter"="Counter", "Ttrigger channels"="Ttrigger channels", "Frequency"="trigger rate 2") -> ("gain task"=w400:refnum<k21>, "sample task"=w401:refnum<k21>, "task out"=w399:refnum<k21>, "SampClk.Rate 2"=→"SampClk.Rate 2":dbl, "Actual Frequency"=→"actual triggere rate":dbl, "error out"=w398:errorcluster)  [unwired: 3 in]
            n175 = while {
              tunnel: w423 -> [w592]
              stop <- w590 stop-if-true
              n176 = Get Queue Status(queue=w592) -> (error out=w590:errorcluster, # elements in queue=w589:i32)  [unwired: 2 in, 6 out]
              n177 = Wait (ms) "Wait"(milliseconds to wait=u32 50) -> ()  [unwired: 1 out]
              n178 = case shown="No Error" w590 {
                tunnel: w589 -> [w593 _]
                frame No Error {
                  "# elements in queue" <- w593
                }
                frame Error {
                }
              }
            }
            n179 = while {
              tunnel: w423 -> [w443]
              tunnel: [w440] -> w420
              tunnel: [w439] -> w419
              tunnel: w413 -> [w438]
              tunnel: w394 -> [w437]
              tunnel: w412 -> [w436]
              tunnel: [w435] -> w396
              tunnel: w382 -> [w434]
              tunnel: w385 -> [w433]
              tunnel: w382 -> [w430]
              stop <- w431 stop-if-true
              n180 = Dequeue Element(queue=w443) -> (element=w442:dbl[], error out=w432:errorcluster)  [unwired: 2 in, 2 out]
              n181 = Equal?(x=w430, y=3.0) -> (x = y?=w428:bool)
              n182 = Wait (ms)(milliseconds to wait="Delay time") -> ()  [unwired: 1 out]
              n183 = Or(x=w432, y=w428) -> (x .or. y?=w431:bool)
              n184 = case shown="No Error" w432 {
                tunnel: w442 -> [w446 _]
                tunnel: [w459 _] -> w440
                tunnel: [w458 _] -> w439
                tunnel: w438 -> [w457 _]
                tunnel: w437 -> [w450 _]
                tunnel: w436 -> [w456 _]
                tunnel: [w447 w587] -> w435
                tunnel: w434 -> [w445 _]
                tunnel: w433 -> [w451 _]
                frame No Error {
                  n185 = call "Sample_process.vi"("Start"="Start", "Frame number"=w450, "Sample data"=w446) -> ("Image date"=w455:dbl[])  [unwired: 8 in]
                  n186 = Initialize Array(0.0 ("element"), w445) -> (w448:dbl[])
                  n187 = for {
                    N: w445 -> [_]
                    tunnel: [w474] -> w459
                    tunnel: [w473] -> w458
                    tunnel: w457 -> [w472]
                    tunnel: w456 -> [w471]
                    tunnel: w455 -> [w469]
                    tunnel: "Auto Swing" -> [w468]
                    tunnel: "Basis 1" -> [w467]
                    tunnel: "Swing 1" -> [w466]
                    tunnel: w451 -> [w465]
                    shift-right: [w462] -> w447
                    shift-left: w448 -> [w464]
                    tunnel: "Image Processing Methods" -> [w461]
                    i -> [w463]
                    n188 = case shown="..0" w463 {
                      tunnel: [w496 w538 w570] -> w474
                      tunnel: [w497 w537 w569] -> w473
                      tunnel: w469 -> [w494 w525 w567]
                      tunnel: w472 -> [w481 w515 w552]
                      tunnel: w471 -> [w480 w514 w551]
                      tunnel: [w487 w523 w558] -> w470
                      tunnel: w468 -> [w491 w529 w563]
                      tunnel: w467 -> [w490 w528 w562]
                      tunnel: w466 -> [w489 w527 w561]
                      tunnel: w465 -> [w492 w524 w564]
                      tunnel: w461 -> [w484 w521 w557]
                      frame ..0 {
                        w499 = u32 4 items=["8 bits", "16 bits", "Float", "Complex", "RGB", "HSL"] ("Image Type")
                        # "Auto compute the middle area's position, then show 300 (or other) points"
                        n189 = Array Subset(array=w494, index=0, length=w492) -> (w477:dbl[])
                        "After oversampling-average 1" <- w477
                        n190 = for {
                          tunnel: w477 -> [w504] mode=indexing
                          shift-right: [w505] -> w478
                          shift-left: 0.0 -> [w506]
                          n191 = Square(x=w504) -> (x^2=w503:dbl)
                          n192 = Add(x=w506, y=w503) -> (x+y=w505:dbl)
                        }
                        "sum sq 1" <- w478
                        n193 = Array Max & Min(array=w477) -> (max value=w476:dbl, min value=→"min value 1":dbl)  [unwired: 2 out]
                        "max value 1" <- w476
                        n194 = call "Contrast_adjust.vi"("Basis"=w490, "Swing voltage"=w489, "Auto adjust"=w491, "Pixel number"=w492, "Modulate date"=w477) -> ("Array"=w485:dbl[])  [unwired: 6 in]
                        n195 = call-poly <vilib>:"Mean.vi"("X"=w477) -> ("mean"=w488:dbl)  [unwired: 1 out]
                        "mean 1" <- w488
                        n196 = Reshape Array(w485, w481, w480) -> (w486:dbl[][])
                        n197 = Reshape Array(w477, w481, w480) -> (w483:dbl[][])
                        n198 = script code="sum =0;\nfor i=2:(X-1)\n    for j= 2:(Y-1)\n        sum = sum +(A(i,j)-A(i-1,j))^2+(A(i,j)-A(i+1,j))^2+(A(i,j)-A(i,j-1))^2+(A(i,j)-A(i,j+1))^2+(A(i,j)-A(i-1,j-1))^2+(A(i,j)-A(i-1,j+1))^2+(A(i,j)-A(i+1,j-1))^2+(A(i,j)-A(i+1,j+1))^2;\n    end\nend\nssum = sqrt(sum)/max"("A"=w483, "X"=w481, "Y"=w480, "max"=w476) -> ("ssum"=w482:dbl, "sum"=w475:dbl)  [unwired: 1 in, 1 out]
                        "diff sq 1" <- w482
                        "1" <- w475
                        n199 = case shown="4.." w484 {
                          tunnel: w488 -> [w507 _ _ _ _]
                          tunnel: [w507 w508 w509 w510 w511] -> w487
                          tunnel: w476 -> [_ w508 _ _ _]
                          tunnel: w482 -> [_ _ _ w510 _]
                          tunnel: w478 -> [_ _ w509 _ _]
                          tunnel: w475 -> [_ _ _ _ w511]
                          frame ..0 {
                          }
                          frame 1 {
                          }
                          frame 2 {
                          }
                          frame 3 {
                          }
                          frame 4.. {
                          }
                        }
                        n200 = Transpose Matrix(1:w486) -> (0:w498:dbl[][])
                        n201 = call "IMAQ Create"("Image Name"="Source 1", "Image Type"=w499) -> ("New Image"=w501:T1, "error out"=w500:errorcluster)  [unwired: 3 in]
                        n202 = call "IMAQ ArrayToColorImage"("Image Pixels (U32)"=w498, "Image"=w501, "error in (no error)"=w500) -> ("Image Out"=w496:T1, "error out"=w497:errorcluster)  [unwired: 2 in]
                        "Frame 1" <- w496
                      }
                      frame 1 {
                        w533 = u32 4 items=["8 bits", "16 bits", "Float", "Complex", "RGB", "HSL"] ("Image Type")
                        # "Auto compute the middle area's position, then show 300 (or other) points"
                        n203 = Array Subset(array=w525, index=w524, length=w524) -> (w516:dbl[])
                        "After oversampling-average 2" <- w516
                        n204 = call "Contrast_adjust.vi"("Basis"=w528, "Swing voltage"=w527, "Auto adjust"=w529, "Pixel number"=w524, "Modulate date"=w516) -> ("Array"=w526:dbl[])  [unwired: 6 in]
                        n205 = Array Max & Min(array=w516) -> (max value=w513:dbl, min value=→"min value 2":dbl)  [unwired: 2 out]
                        "max value 2" <- w513
                        n206 = call-poly <vilib>:"Mean.vi"("X"=w516) -> ("mean"=w522:dbl)  [unwired: 1 out]
                        "mean 2" <- w522
                        n207 = for {
                          tunnel: w516 -> [w540] mode=indexing
                          shift-right: [w541] -> w519
                          shift-left: 0.0 -> [w542]
                          n208 = Square(x=w540) -> (x^2=w539:dbl)
                          n209 = Add(x=w542, y=w539) -> (x+y=w541:dbl)
                        }
                        "sq sum 2" <- w519
                        n210 = Reshape Array(w516, w515, w514) -> (w518:dbl[][])
                        n211 = Reshape Array(w526, w515, w514) -> (w531:dbl[][])
                        n212 = script code="sum =0;\nfor i=2:(X-1)\n    for j= 2:(Y-1)\n        sum = sum +(A(i,j)-A(i-1,j))^2+(A(i,j)-A(i+1,j))^2+(A(i,j)-A(i,j-1))^2+(A(i,j)-A(i,j+1))^2+(A(i,j)-A(i-1,j-1))^2+(A(i,j)-A(i-1,j+1))^2+(A(i,j)-A(i+1,j-1))^2+(A(i,j)-A(i+1,j+1))^2;\n    end\nend\n\nssum = sqrt(sum)/max;"("A"=w518, "X"=w515, "Y"=w514, "max"=w513) -> ("ssum"=w517:dbl, "sum"=w512:dbl)  [unwired: 1 in, 1 out]
                        "diff sq 2" <- w517
                        "2" <- w512
                        n213 = case shown="4" w521 {
                          tunnel: w522 -> [w543 _ _ _ _]
                          tunnel: [w543 w544 w545 w546 w547] -> w523
                          tunnel: w513 -> [_ w544 _ _ _]
                          tunnel: w519 -> [_ _ w545 _ _]
                          tunnel: w517 -> [_ _ _ w546 _]
                          tunnel: w512 -> [_ _ _ _ w547]
                          frame ..0, Default {
                          }
                          frame 1 {
                          }
                          frame 2 {
                          }
                          frame 3 {
                          }
                          frame 4 {
                          }
                        }
                        n214 = Transpose Matrix(1:w531) -> (0:w532:dbl[][])
                        n215 = call "IMAQ Create"("Image Name"="Source 1", "Image Type"=w533) -> ("New Image"=w535:T1, "error out"=w534:errorcluster)  [unwired: 3 in]
                        n216 = call "IMAQ ArrayToColorImage"("Image Pixels (U32)"=w532, "Image"=w535, "error in (no error)"=w534) -> ("Image Out"=w538:T1, "error out"=w537:errorcluster)  [unwired: 2 in]
                        "Frame 2" <- w538
                      }
                      frame 2.. {
                        w573 = u32 4 items=["8 bits", "16 bits", "Float", "Complex", "RGB", "HSL"] ("Image Type")
                        # "Auto compute the middle area's position, then show 300 (or other) points"
                        n217 = Multiply(x=2.0, y=w564) -> (x*y=w565:dbl)
                        n218 = Array Subset(array=w567, index=w565, length=w564) -> (w553:dbl[])
                        "After oversampling-average 3" <- w553
                        n219 = for {
                          tunnel: w553 -> [w578] mode=indexing
                          shift-right: [w579] -> w555
                          shift-left: 0.0 -> [w580]
                          n220 = Square(x=w578) -> (x^2=w577:dbl)
                          n221 = Add(x=w580, y=w577) -> (x+y=w579:dbl)
                        }
                        "sum sq 3" <- w555
                        n222 = call "Contrast_adjust.vi"("Basis"=w562, "Swing voltage"=w561, "Auto adjust"=w563, "Pixel number"=w564, "Modulate date"=w553) -> ("Array"=w560:dbl[])  [unwired: 6 in]
                        n223 = Array Max & Min(array=w553) -> (max value=w549:dbl, min value=→"min value 3":dbl)  [unwired: 2 out]
                        "max value 3" <- w549
                        n224 = call-poly <vilib>:"Mean.vi"("X"=w553) -> ("mean"=w559:dbl)  [unwired: 1 out]
                        "mean 3" <- w559
                        n225 = Reshape Array(w560, w552, w551) -> (w571:dbl[][])
                        n226 = Reshape Array(w553, w552, w551) -> (w554:dbl[][])
                        n227 = script code="sum =0;\nfor i=2:(X-1)\n    for j= 2:(Y-1)\n        sum = sum +(A(i,j)-A(i-1,j))^2+(A(i,j)-A(i+1,j))^2+(A(i,j)-A(i,j-1))^2+(A(i,j)-A(i,j+1))^2+(A(i,j)-A(i-1,j-1))^2+(A(i,j)-A(i-1,j+1))^2+(A(i,j)-A(i+1,j-1))^2+(A(i,j)-A(i+1,j+1))^2;\n    end\nend\n\nssum = sqrt(sum)/max;"("A"=w554, "X"=w552, "Y"=w551, "max"=w549) -> ("ssum"=w550:dbl, "sum"=w548:dbl)  [unwired: 1 in, 1 out]
                        "diff sq 3" <- w550
                        "3" <- w548
                        n228 = case shown="4.." w557 {
                          tunnel: w559 -> [w581 _ _ _ _]
                          tunnel: [w581 w582 w583 w584 w585] -> w558
                          tunnel: w549 -> [_ w582 _ _ _]
                          tunnel: w555 -> [_ _ w583 _ _]
                          tunnel: w550 -> [_ _ _ w584 _]
                          tunnel: w548 -> [_ _ _ _ w585]
                          frame ..0, Default {
                          }
                          frame 1 {
                          }
                          frame 2 {
                          }
                          frame 3 {
                          }
                          frame 4.. {
                          }
                        }
                        n229 = Transpose Matrix(1:w571) -> (0:w572:dbl[][])
                        n230 = call "IMAQ Create"("Image Name"="Source 1", "Image Type"=w573) -> ("New Image"=w575:T1, "error out"=w574:errorcluster)  [unwired: 3 in]
                        n231 = call "IMAQ ArrayToColorImage"("Image Pixels (U32)"=w572, "Image"=w575, "error in (no error)"=w574) -> ("Image Out"=w570:T1, "error out"=w569:errorcluster)  [unwired: 2 in]
                        "Frame 3" <- w570
                      }
                    }
                    n232 = Replace Array Subset(array=w464, new element=w470, index=w463) -> (w462:dbl[])
                  }
                  "Raw Data" <- w446
                }
                frame Error {
                  n233 = Initialize Array(0.0 ("element"), 1 ("dimension size")) -> (w587:dbl[])
                }
              }
            }
            n234 = while {
              shift-right: [w621] -> w425
              shift-left: w427 -> [w622]
              shift-right: [w623] -> w426
              shift-left: w423 -> [w624]
              tunnel: w401 -> [w620]
              tunnel: w398 -> [w619]
              tunnel: w410 -> [w618]
              tunnel: [w617] -> w422
              tunnel: w399 -> [w614]
              tunnel: [w612] -> w418
              tunnel: [w611] -> w417
              tunnel: [w605] -> _
              tunnel: [w606] -> w415
              tunnel: w400 -> [w605]
              tunnel: [w598] -> w384
              i -> [w596]
              stop <- w598 continue-if-true
              n235 = Equal To 0?(x=w596) -> (x = 0?=w594:bool)
              n236 = call-poly <vilib>:"DAQmx Read.vi"("task/channels in"=w620, "number of samples per channel"=w618, "timeout"=10.0, "error in"=w619) -> ("task out"=w617:refnum<k21>, "data"=w595:dbl[], "error out"=w613:errorcluster)  [unwired: 9 in]
              n237 = Multiply(x=0.036, y="Gain_Ch0") -> (x*y=w607:dbl)
              n238 = case shown="True" w594 {
                tunnel: w595 -> [_ w625]
                frame False {
                }
                frame True {
                  "Array" <- w625
                }
              }
              n239 = local read "Wavefront Correction"() -> (w601:bool)
              n240 = local read "# elements in queue"() -> (w616:i32)
              n241 = case shown="True" TRUE {
                tunnel: w624 -> [w627 w632]
                tunnel: [w627 w631] -> w623
                tunnel: w622 -> [w626 w630]
                tunnel: [w626 w629] -> w621
                tunnel: w595 -> [_ w628]
                frame False {
                }
                frame True {
                  n242 = Enqueue Element(queue=w632, element=w628, error in (no error)=w630) -> (queue out=w631:refnum<queue>, error out=w629:errorcluster)  [unwired: 1 in, 1 out]
                }
              }
              n243 = call-poly <vilib>:"DAQmx Write.vi"("task/channels in"=w605, "data"=w607) -> ("task out"=w606:refnum<k21>)  [unwired: 11 in, 2 out]
              n244 = Not(x=w601) -> (.not. x?=w597:bool)
              n245 = Not(x="Stop Imaging") -> (.not. x?=w602:bool)
              n246 = Less?(x=w616, y=100) -> (x < y?=w604:bool)
              n247 = And(x=w602, y=w604) -> (x .and. y?=w600:bool)
              n248 = And(x=w597, y=w600) -> (x .and. y?=w598:bool)
              n249 = call <vilib>:"DAQmx Is Task Done.vi"("task/channels in"=w614, "error in"=w613) -> ("task out"=w612:refnum<k21>, "error out"=w611:errorcluster)  [unwired: 11 in, 1 out]
            }
            n250 = Release Queue(queue=w426, error in (no error)=w425) -> ()  [unwired: 1 in, 3 out]
            n251 = call <vilib>:"DAQmx Clear Task.vi"("task in"=w418, "error in"=w417) -> ("error out"=w416:errorcluster)  [unwired: 13 in]
            n252 = call <vilib>:"DAQmx Clear Task.vi"("task in"=w422, "error in"=w416) -> ("error out"=w414:errorcluster)  [unwired: 13 in]
            n253 = call "IMAQ Dispose"("Image"=w420, "error in (no error)"=w419) -> ()  [unwired: 4 in, 1 out]
            "Imaging" <- TRUE
          }
          frame #1 {
            # "Must set the gain output to 0 volts before stopping the program"
            n254 = Not(x=w635) -> (.not. x?=w634:bool)
            n255 = local read "Wavefront Correction"() -> (w637:bool)
            n256 = case shown="True" w634 {
              tunnel: w646 -> [w675 w680]
              tunnel: [w675 w678] -> w644
              tunnel: [w674 w677] -> w643
              tunnel: w645 -> [w674 w681]
              frame False {
              }
              frame True {
                n257 = dll-call lib="D:/documents/Dropbox/Only me/wavefront_correction/LabVIEW Control Codes/LabVIEW Codes/alp4395.dll" fn="AlpProjHalt"(path in=w680, "DeviceId"=w681) -> (path out=w679:path, "DeviceId"=w676:u32)  [unwired: 3 in, 1 out]
                n258 = dll-call lib="D:/documents/Dropbox/Only me/wavefront_correction/LabVIEW Control Codes/LabVIEW Codes/alp4395.dll" fn="AlpDevHalt"(path in=w679, "DeviceId"=w676) -> (path out=w678:path, "DeviceId"=w677:u32)  [unwired: 3 in, 1 out]
              }
            }
            n259 = case shown="True" w637 {
              tunnel: w642 -> [_ w663]
              tunnel: [w655 w661] -> w641
              tunnel: [w654 w660] -> w640
              tunnel: w639 -> [w654 w659]
              tunnel: w638 -> [w655 w658]
              tunnel: [T2."Idle" T2."Free pics"] -> w636
              frame False {
              }
              frame True {
                n260 = Array Max & Min(array=w663) -> (max index (indices)=w662:i32)  [unwired: 3 out]
                "max index" <- w662
                n261 = case shown="..0" w662 {
                  tunnel: w658 -> [w665 w670 w672]
                  tunnel: [w665 w668 w672] -> w661
                  tunnel: [w664 w667 w671] -> w660
                  tunnel: w659 -> [w666 w667 w673]
                  frame ..0 {
                    n262 = Subtract(x=w666, y=w665) -> (x-y=w664:dbl)
                  }
                  frame 1 {
                    n263 = Divide(x=w670, y=2.0) -> (x/y=w668:dbl)
                  }
                  frame 2.. {
                    n264 = Add(x=w673, y=w672) -> (x+y=w671:dbl)
                  }
                }
                n265 = call "Servo Control-780nm_WC.vi"("DMD Shutter"=FALSE) -> ()  [unwired: 11 in]
                "evaluation value" <- w663
              }
            }
            "Real time search gap" <- w641
            "Real time Centre A" <- w640
            n266 = local write "Hill-climbing \n   finished"(FALSE ("Hill-climbing \n   finished")) -> ()
            n267 = call-poly <vilib>:"DAQmx Write.vi"("task/channels in"=w647, "data"=0.0, "error in"=w648) -> ("task out"=w651:refnum<k21>, "error out"=w650:errorcluster)  [unwired: 10 in, 1 out]
            n268 = call <vilib>:"DAQmx Clear Task.vi"("task in"=w651, "error in"=w650) -> ("error out"=→"Error Out":errorcluster)  [unwired: 13 in]
          }
        }
      }
      frame "Free pics".. {
        # "SeqFree"
        n269 = dll-call lib="?" fn="AlpSeqFree"(path in=w696, "DeviceId"=w695, "SequenceId"=w694) -> (path out=w693:path, "DeviceId"=w691:u32, "SequenceId"=w692:u32)  [unwired: 3 in, 1 out]
        n270 = local write "Free pics"(FALSE ("Free pics")) -> ()
        n271 = local read "Wavefront Correction"() -> (w687:bool)
        n272 = Select(t=T2."Idle", s=w687, f=T2."No sequence") -> (s? t:f=w686:T2)
      }
    }
  }
  n273 = flat-sequence {
    tunnel: w10 -> [w701]
    tunnel: w9 -> [w700]
    tunnel: w8 -> [w697]
    frame #0 {
      # "ProjHalt"
      # "SeqFree"
      # "DevFree"
      n274 = dll-call lib="?" fn="AlpProjHalt"(path in=w701, "DeviceId"=w700) -> (path out=w698:path, "DeviceId"=w699:u32)  [unwired: 3 in, 1 out]
      n275 = dll-call lib="?" fn="AlpSeqFree"(path in=w698, "DeviceId"=w699, "SequenceId"=w697) -> (path out=w703:path, "DeviceId"=w702:u32)  [unwired: 4 in, 1 out]
      n276 = dll-call lib="?" fn="AlpDevFree"(path in=w703, "DeviceId"=w702) -> ()  [unwired: 4 in, 2 out]
    }
  }
